vi "Self-Test.vi"(6 "Remote Timeout (300,000 ms)":u32=300000, 8 "error in (no error)":errorcluster, 9 "Prompt if Full Mode (T)":bool=TRUE, 10 "Self-Test Mode (basic)":i32(ring) items=["basic", "intermediate", "full"], 11 "Resource in":refnum<k20>) -> (0 "error out":errorcluster, 2 "Detailed Result":string, 3 "Resource out":refnum<k20>)   [LabVIEW 2020, in "nisyscfg.lvlib"]
doc: "Verifies that system devices can perform basic I/O functions. Ensure that no other tasks are running on the system while the self-test executes because the driver may need exclusive access to some device resources.\n\nYou can select from three modes that provide different levels of self-test functionality. The mode you select might require you to disconnect cables from the device. For details about each mode, refer to the description for the <B>Self-Test Mode</B> input."
uses:
  <vilib>/nisyscfg/nisyscfg.lvlib
  <vilib>/Utility/error.llb/Error Cluster From Error Code.vi
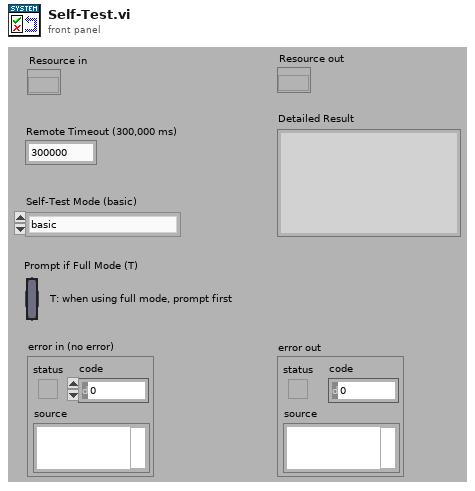
[diagram p1: front panel]
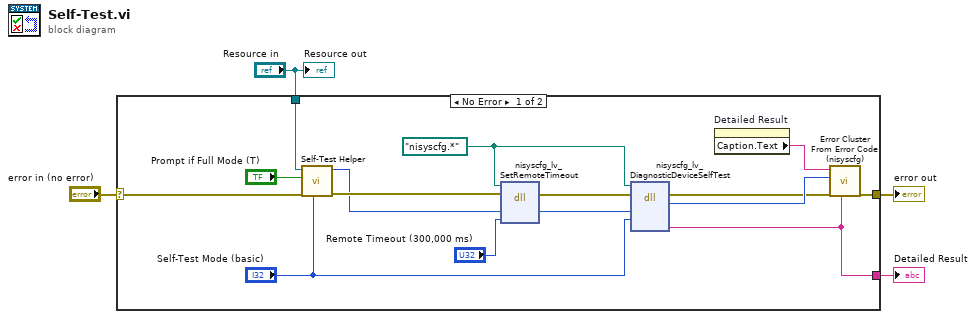
[diagram p0: block diagram]
diagram:
  n1 = case shown="No Error" "error in (no error)" {
    selector: "error in (no error)" -> [w10 w20]
    tunnel: [w17 w20] -> w4
    tunnel: "Resource in" -> [w5 _]
    tunnel: [w11 _] -> w1
    frame No Error {
      w13 = path "nisyscfg.*" ("path in")
      n2 = call <vilib>:"Self-Test Helper.vi"("Self-Test Mode (basic)"="Self-Test Mode (basic)", "error in (no error)"=w10, "Prompt if Full Mode (T)"="Prompt if Full Mode (T)", "Resource in"=w5) -> ("error out"=w7:errorcluster, "Resource out"=w6:u64)  [unwired: 6 in]
      n3 = dll-call lib="nisyscfg.*" fn="nisyscfg_lv_SetRemoteTimeout" label="SetRemoteTimeout"(path in=w13, error in=w7, "item"=w6, "connectTimeout"="Remote Timeout (300,000 ms)") -> (error out=w16:errorcluster, "item"=w14:u64)  [unwired: 1 in, 3 out]
      n4 = dll-call lib="nisyscfg.*" fn="nisyscfg_lv_DiagnosticDeviceSelfTest" label="DiagnosticDeviceSelfTest"(path in=w13, error in=w16, "item"=w14, "mode"="Self-Test Mode (basic)") -> (error out=w18:errorcluster, "status"=w19:i32, "detailed result"=w11:string)  [unwired: 2 in, 3 out]
      n5 = property on="Detailed Result" class="Str"() -> ("Caption.Text"=w12:string)  [unwired: 2 in, 2 out]
      n6 = call <vilib>:"Error Cluster From Error Code (nisyscfg).vi"("Details String"=w11, "error in (no error)"=w18, "Error Code (0)"=w19, "Details Caption"=w12) -> ("error out"=w17:errorcluster)  [unwired: 7 in]
    }
    frame Error {
    }
  }
  "error out" <- w4
  "Detailed Result" <- w1
  "Resource out" <- "Resource in"
